vi "PedalDigital.vi"() -> ()   [LabVIEW 2013]
uses:
  <vilib>/express/express analysis/Spectral/Block/exnSpectralBlock spectral measurements RMS poly.vi
  <vilib>/express/express analysis/Spectral/Block/exnSpectralBlock spectral measurements RMS WFM.vi
  <vilib>/express/express analysis/Spectral/XNode/ExpressSpectralMeasurementsBlockNode.xnode
  <vilib>/measure/NI_MABase.lvlib
panel:
  out "Digital signal":dbl[](graph)
  in  "stop":bool
  in  "Gain":dbl(slide)=1.0 scale=0.0..1.0
  in  "Tone":dbl(slide) scale=10.0..100.0
  in  "Distortion":dbl(slide)=1.0 scale=0.0..4000.0
  out "Distorted Signal":waveform(dbl)(graph)
  out "FFT":cluster{"f0":dbl, "df":dbl, "magnitude":dbl[]}(graph)
  out "Clean Signal":waveform(dbl)(graph)
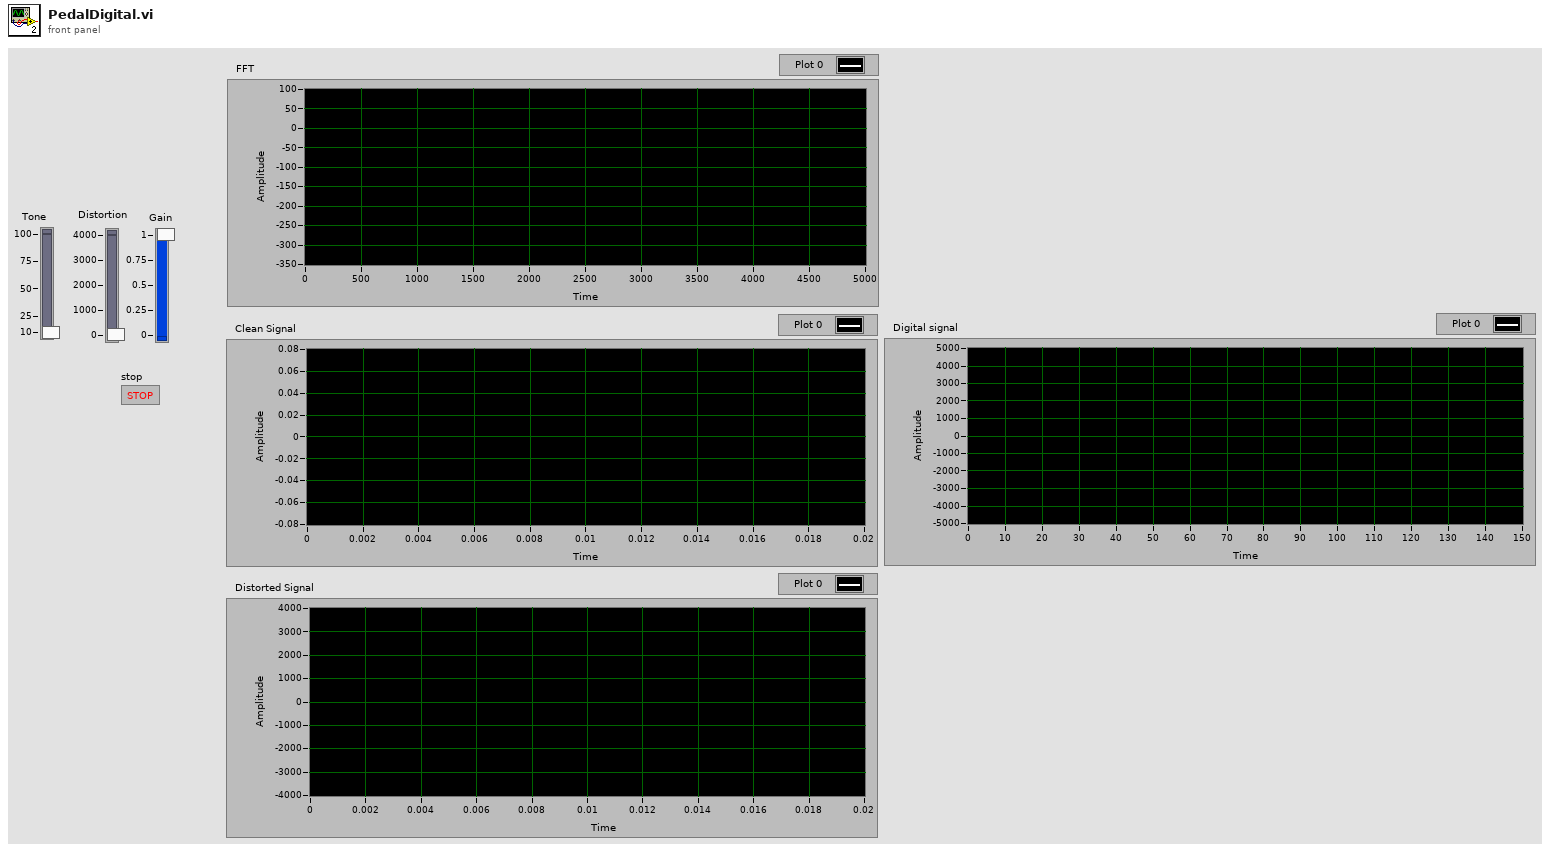
[diagram p1: front panel]
types:
  T1 = cluster{"averaging mode":u16, "weighting mode":u16, "number of averages":u32}
  T2 = cluster{"dB On (F)":bool, "unwrap phase (F)":bool, "convert to degree (F)":bool}
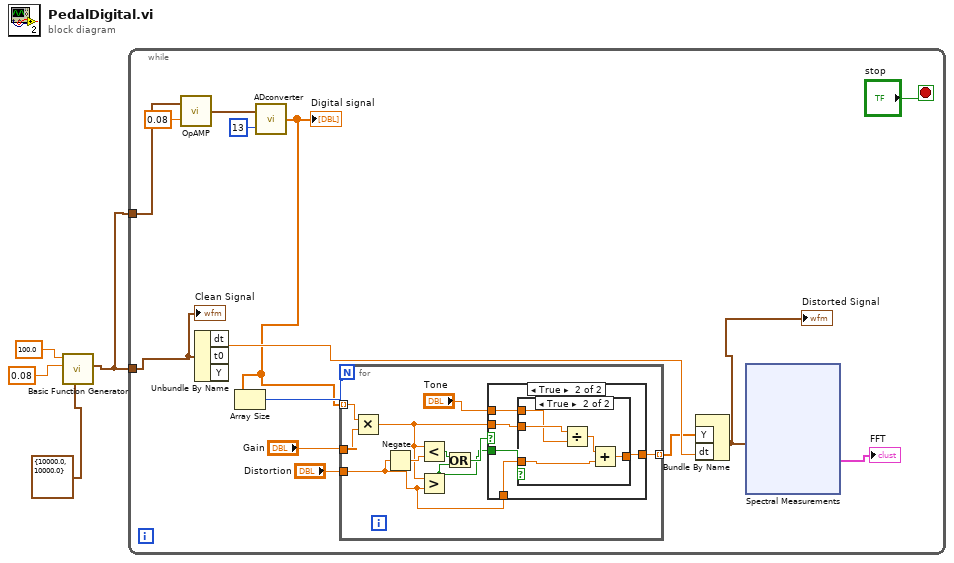
[diagram p0: block diagram]
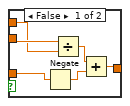
[diagram p3: hidden frame]
diagram:
  n1 = call <vilib>:"Basic Function Generator.vi"("sampling info"=cluster{"#s":dbl, "Fs":dbl} {"#s"=10000.0, "Fs"=10000.0}, "amplitude"=0.08, "frequency"=100.0) -> ("signal out"=w1:waveform(dbl))  [unwired: 6 in, 2 out]
  n2 = while {
    tunnel: w1 -> [w11]
    tunnel: w1 -> [w8]
    stop <- "stop" stop-if-true
    n3 = call "OpAMP.vi"("Max Amplitude"=0.08, "Analog Signal"=w8) -> ("Amplified signal"=w6:waveform(dbl))
    n4 = Unbundle By Name(w11) -> ("dt"=w15:dbl)  [unwired: 2 out]
    n5 = call "ADconverter.vi"("resolution (16 bit)"=13, "Analog signal"=w6) -> ("Digital signal"=w5:dbl[])
    "Digital signal" <- w5
    n6 = Array Size(array=w5) -> (size(s)=w16:i32)
    n7 = for {
      N: w16 -> [_]
      tunnel: w5 -> [w37] mode=indexing
      tunnel: "Gain" -> [w38]
      tunnel: "Distortion" -> [w35]
      tunnel: [w36] -> w13 mode=indexing
      n8 = Multiply(x=w37, y=w38) -> (x*y=w33:dbl)
      n9 = Negate(x=w35) -> (-x=w34:dbl)
      n10 = Less?(x=w33, y=w34) -> (x < y?=w31:bool)
      n11 = Greater?(x=w33, y=w35) -> (0:w30:bool)
      n12 = Or(x=w31, y=w30) -> (x .or. y?=w32:bool)
      n13 = case shown="True" w32 {
        tunnel: [w39 w41] -> w36
        tunnel: w33 -> [w39 w44]
        tunnel: w35 -> [_ w43]
        tunnel: w30 -> [_ w42]
        tunnel: "Tone" -> [_ w40]
        frame False {
        }
        frame True {
          n14 = case shown="True" w42 {
            tunnel: w44 -> [w46 w52]
            tunnel: w43 -> [w47 w53]
            tunnel: [w49 w54] -> w41
            tunnel: w40 -> [w45 w51]
            frame False {
              n15 = Negate(x=w47) -> (-x=w48:dbl)
              n16 = Divide(x=w46, y=w45) -> (x/y=w50:dbl)
              n17 = Add(x=w50, y=w48) -> (x+y=w49:dbl)
            }
            frame True {
              n18 = Divide(x=w52, y=w51) -> (x/y=w55:dbl)
              n19 = Add(x=w55, y=w53) -> (x+y=w54:dbl)
            }
          }
        }
      }
    }
    n20 = Bundle By Name("Y"=w13, "dt"=w15) -> (w9:waveform(dbl))  [unwired: 1 in]
    "Distorted Signal" <- w9
    n21 = xnode "Spectral Measurements"("Signals"=w9) -> ("FFT - (RMS)"=→"FFT":cluster{"f0":dbl, "df":dbl, "magnitude":dbl[]})  [unwired: 1 in, 2 out]
    "Clean Signal" <- w11
  }
